vi "Save data file (pass-fail) v5.vi"(8 "Input Cluster":T1, 11 "panel id":string) -> (0 "network file save error":errorcluster, 3 "file save path":string)   [LabVIEW 2017]
uses:
  Global 1.vi
  Global display 2.vi
  Global display 3.vi
  <vilib>/Utility/file.llb/Write Delimited Spreadsheet (string).vi
panel:
  out "Fail File path":path
  out "x != y?":bool
  out "mail file":bool
  out "Report path c drive":path
  out "Report path network":path
  out "status":string
  out "C drive root path":string
  out "network file dir path":path
  out "network dir":string
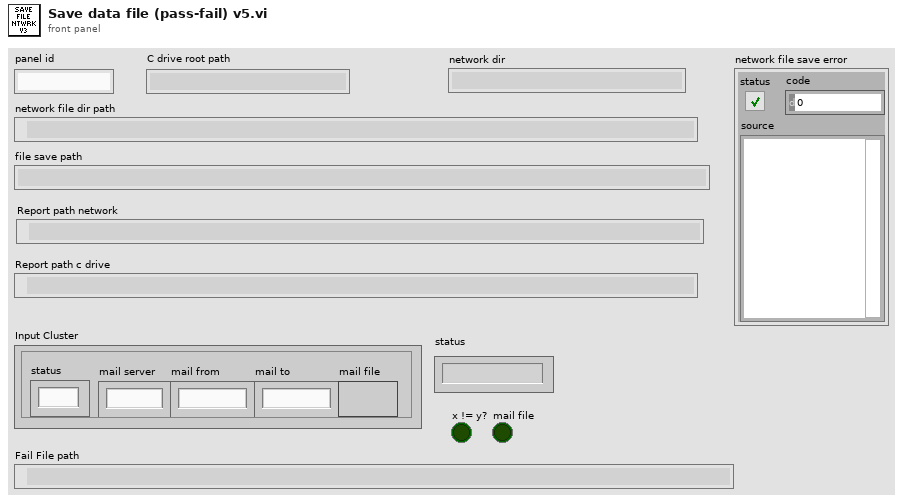
[diagram p1: front panel]
types:
  T1 = cluster{"status":string, "mail server":string, "mail from":string, "mail to":string, "mail file":bool}
  T2 = cluster{"CYCLE":dbl, "MINS":dbl, "STATUS":string}
  T3 = cluster{"NAME":string, "DESCRIPTION":string, "CYCLES":dbl, "T-RISE mins":dbl, "T-RISE deg C":dbl}
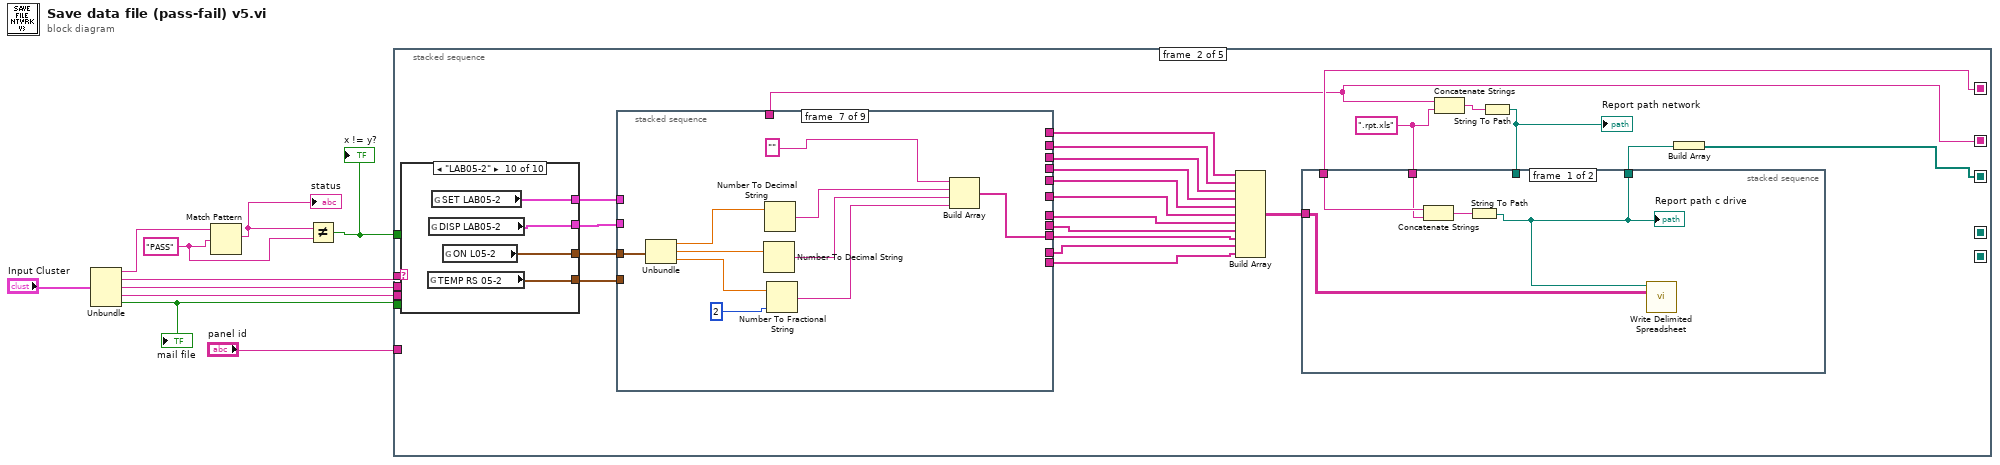
[diagram p0: block diagram]
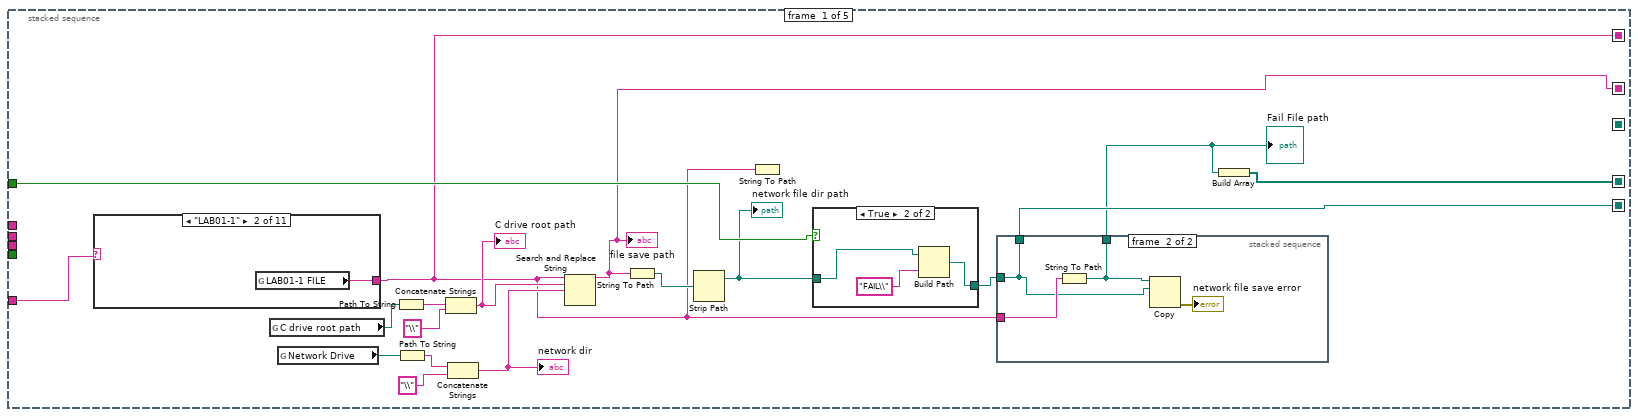
[diagram p2: hidden frame]
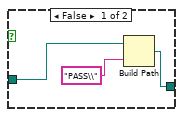
[diagram p3: hidden frame]
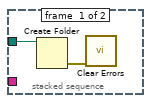
[diagram p4: hidden frame]
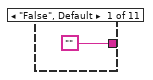
[diagram p5: hidden frame]
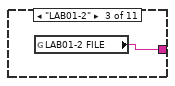
[diagram p6: hidden frame]
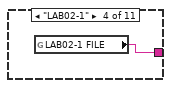
[diagram p7: hidden frame]
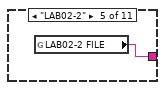
[diagram p8: hidden frame]
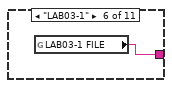
[diagram p9: hidden frame]
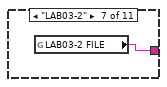
[diagram p10: hidden frame]
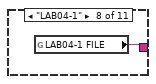
[diagram p11: hidden frame]
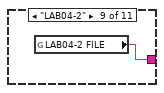
[diagram p12: hidden frame]
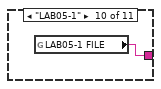
[diagram p13: hidden frame]
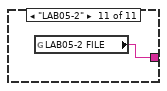
[diagram p14: hidden frame]
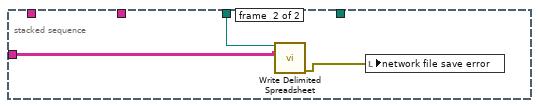
[diagram p15: hidden frame]
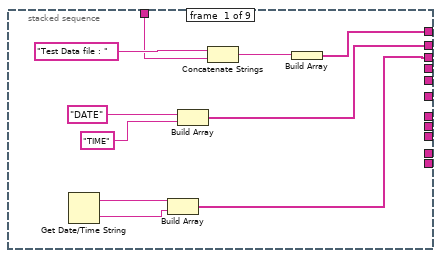
[diagram p16: hidden frame]
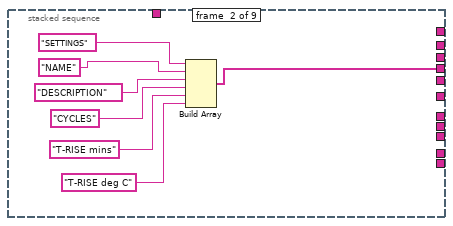
[diagram p17: hidden frame]
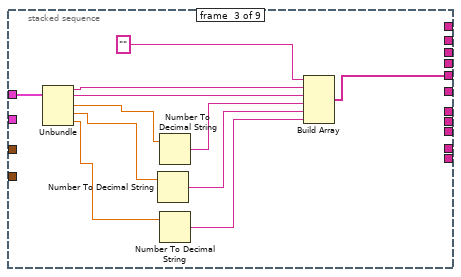
[diagram p18: hidden frame]
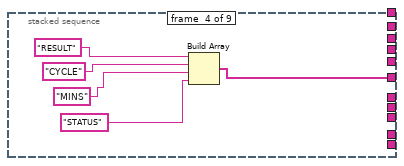
[diagram p19: hidden frame]
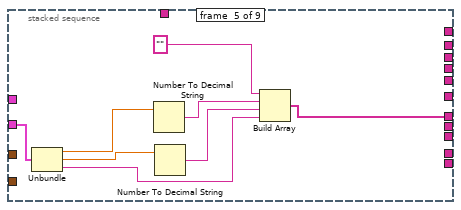
[diagram p20: hidden frame]
diagram:
  w10 = "PASS"
  n1 = Unbundle("Input Cluster") -> ("status"=w8:string, "mail server"=w2:string, "mail from"=w3:string, "mail to"=w4:string, "mail file"=w5:bool)
  "mail file" <- w5
  n2 = Match Pattern(string=w8, regular expression=w10) -> (match substring=w9:string)  [unwired: 1 in, 3 out]
  "status" <- w9
  n3 = Not Equal?(x=w9, y=w10) -> (x != y?=w6:bool)
  "x != y?" <- w6
  n4 = stacked-sequence {
    seq-local: [w11 _ _ _ _] -> [_ _ _ w197 _]
    seq-local: [w17 _ _ _ _] -> [_ _ _ _ _]
    seq-local: [w16 _ _ _ _] -> [_ w53 _ _ _]
    seq-local: [_ w56 _ _ _] -> [_ _ _ _ w207]
    seq-local: [w13 _ _ _ _] -> [_ w55 _ _ _]
    tunnel: w6 -> [w20 _ _ w196 _]
    tunnel: w5 -> [_ _ _ w195 _]
    tunnel: w4 -> [_ _ _ w194 _]
    tunnel: w3 -> [_ _ _ w193 w209]
    tunnel: w2 -> [_ _ _ w192 w208]
    tunnel: "panel id" -> [w15 w70 _ _ _]
    frame #0 {
      n5 = case shown="\"LAB01-1\"" w15 {
        tunnel: ["" w42 w43 w44 w45 w46 w47 w48 w49 w50 w51] -> w13
        frame "False", Default {
        }
        frame "LAB01-1" {
          n6 = global read "Global 1.vi" "LAB01-1 FILE"() -> (w42:string)
        }
        frame "LAB01-2" {
          n7 = global read "Global 1.vi" "LAB01-2 FILE"() -> (w43:string)
        }
        frame "LAB02-1" {
          n8 = global read "Global 1.vi" "LAB02-1 FILE"() -> (w44:string)
        }
        frame "LAB02-2" {
          n9 = global read "Global 1.vi" "LAB02-2 FILE"() -> (w45:string)
        }
        frame "LAB03-1" {
          n10 = global read "Global 1.vi" "LAB03-1 FILE"() -> (w46:string)
        }
        frame "LAB03-2" {
          n11 = global read "Global 1.vi" "LAB03-2 FILE"() -> (w47:string)
        }
        frame "LAB04-1" {
          n12 = global read "Global 1.vi" "LAB04-1 FILE"() -> (w48:string)
        }
        frame "LAB04-2" {
          n13 = global read "Global 1.vi" "LAB04-2 FILE"() -> (w49:string)
        }
        frame "LAB05-1" {
          n14 = global read "Global 1.vi" "LAB05-1 FILE"() -> (w50:string)
        }
        frame "LAB05-2" {
          n15 = global read "Global 1.vi" "LAB05-2 FILE"() -> (w51:string)
        }
      }
      n16 = global read "Global 1.vi" "C drive root path"() -> (w22:path)
      n17 = global read "Global 1.vi" "Network Drive"() -> (w28:path)
      n18 = Path To String(path=w22) -> (string=w23:string)
      n19 = Path To String(path=w28) -> (string=w27:string)
      n20 = Concatenate Strings(w23, "\\") -> (w21:string)
      "C drive root path" <- w21
      n21 = Concatenate Strings(w27, "\\") -> (w25:string)
      "network dir" <- w25
      n22 = Search and Replace String(input string=w13, search string=w21, replace string=w25) -> (result string=w16:string)  [unwired: 5 in, 3 out]
      "file save path" <- w16
      n23 = String To Path(string=w16) -> (path=w14:path)
      n24 = Strip Path(path=w14) -> (stripped path=w18:path)  [unwired: 1 out]
      "network file dir path" <- w18
      n25 = String To Path(string=w13) -> ()  [unwired: 1 out]
      n26 = case shown="True" w20 {
        tunnel: [w29 w34] -> w19
        tunnel: w18 -> [w30 w32]
        frame False {
          n27 = Build Path(base path=w30, name or relative path="PASS\\") -> (appended path=w29:path)
        }
        frame True {
          n28 = Build Path(base path=w32, name or relative path="FAIL\\") -> (appended path=w34:path)
        }
      }
      n29 = stacked-sequence {
        tunnel: w19 -> [w36 w38]
        tunnel: w13 -> [_ w39]
        tunnel: [_ w38] -> w17
        tunnel: [_ w37] -> w12
        frame #0 {
          n30 = Create Folder(path (use dialog)=w36) -> (error out=w35:errorcluster)  [unwired: 2 in, 2 out]
          n31 = call <vilib>:"Clear Errors.vi"("error in (no error)"=w35) -> ()  [unwired: 5 in, 2 out]
        }
        frame #1 {
          n32 = String To Path(string=w39) -> (path=w37:path)
          n33 = Copy(10:w38, 11:w37) -> (0:→"network file save error":errorcluster)  [unwired: 3 in, 2 out]
        }
      }
      "Fail File path" <- w12
      n34 = Build Array(w12) -> (w11:path[])
    }
    frame #1 {
      w54 = ".rpt.xls"
      n35 = case shown="\"LAB05-2\"" w70 {
        tunnel: [w154 w158 w162 w166 w170 w174 w178 w182 w186 w190] -> w75
        tunnel: [w153 w157 w161 w165 w169 w173 w177 w181 w185 w189] -> w74
        tunnel: [w152 w156 w160 w164 w168 w172 w176 w180 w184 w188] -> w73
        tunnel: [w151 w155 w159 w163 w167 w171 w175 w179 w183 w187] -> w72
        frame "LAB01-1", Default {
          n36 = global read "Global display 3.vi" "TEMP RS 01-1"() -> (w151:cluster{"TL":dbl, "TN":dbl})
          n37 = global read "Global display 2.vi" "DISP LAB01-1"() -> (w153:T2)
          n38 = global read "Global display 2.vi" "SET LAB01-1"() -> (w154:T3)
          n39 = global read "Global display 2.vi" "ON L01-1"() -> (w152:cluster{"amps":dbl, "volts":dbl, "pf":dbl})
        }
        frame "LAB01-2" {
          n40 = global read "Global display 3.vi" "TEMP RS 01-2"() -> (w155:cluster{"TL":dbl, "TN":dbl})
          n41 = global read "Global display 2.vi" "DISP LAB01-2"() -> (w157:T2)
          n42 = global read "Global display 2.vi" "SET LAB01-2"() -> (w158:T3)
          n43 = global read "Global display 2.vi" "ON L01-2"() -> (w156:cluster{"amps":dbl, "volts":dbl, "pf":dbl})
        }
        frame "LAB02-1" {
          n44 = global read "Global display 3.vi" "TEMP RS 02-1"() -> (w159:cluster{"TL":dbl, "TN":dbl})
          n45 = global read "Global display 2.vi" "DISP LAB02-1"() -> (w161:T2)
          n46 = global read "Global display 2.vi" "SET LAB02-1"() -> (w162:T3)
          n47 = global read "Global display 2.vi" "ON L02-1"() -> (w160:cluster{"amps":dbl, "volts":dbl, "pf":dbl})
        }
        frame "LAB02-2" {
          n48 = global read "Global display 3.vi" "TEMP RS 02-2"() -> (w163:cluster{"TL":dbl, "TN":dbl})
          n49 = global read "Global display 2.vi" "DISP LAB02-2"() -> (w165:T2)
          n50 = global read "Global display 2.vi" "SET LAB02-2"() -> (w166:T3)
          n51 = global read "Global display 2.vi" "ON L02-2"() -> (w164:cluster{"amps":dbl, "volts":dbl, "pf":dbl})
        }
        frame "LAB03-1" {
          n52 = global read "Global display 3.vi" "TEMP RS 03-1"() -> (w167:cluster{"TL":dbl, "TN":dbl})
          n53 = global read "Global display 2.vi" "DISP LAB03-1"() -> (w169:T2)
          n54 = global read "Global display 2.vi" "SET LAB03-1"() -> (w170:T3)
          n55 = global read "Global display 2.vi" "ON L03-1"() -> (w168:cluster{"amps":dbl, "volts":dbl, "pf":dbl})
        }
        frame "LAB03-2" {
          n56 = global read "Global display 3.vi" "TEMP RS 03-2"() -> (w171:cluster{"TL":dbl, "TN":dbl})
          n57 = global read "Global display 2.vi" "DISP LAB03-2"() -> (w173:T2)
          n58 = global read "Global display 2.vi" "SET LAB03-2"() -> (w174:T3)
          n59 = global read "Global display 2.vi" "ON L03-2"() -> (w172:cluster{"amps":dbl, "volts":dbl, "pf":dbl})
        }
        frame "LAB04-1" {
          n60 = global read "Global display 3.vi" "TEMP RS 04-1"() -> (w175:cluster{"TL":dbl, "TN":dbl})
          n61 = global read "Global display 2.vi" "DISP LAB04-1"() -> (w177:T2)
          n62 = global read "Global display 2.vi" "SET LAB04-1"() -> (w178:T3)
          n63 = global read "Global display 2.vi" "ON L04-1"() -> (w176:cluster{"amps":dbl, "volts":dbl, "pf":dbl})
        }
        frame "LAB04-2" {
          n64 = global read "Global display 3.vi" "TEMP RS 04-2"() -> (w179:cluster{"TL":dbl, "TN":dbl})
          n65 = global read "Global display 2.vi" "DISP LAB04-2"() -> (w181:T2)
          n66 = global read "Global display 2.vi" "SET LAB04-2"() -> (w182:T3)
          n67 = global read "Global display 2.vi" "ON L04-2"() -> (w180:cluster{"amps":dbl, "volts":dbl, "pf":dbl})
        }
        frame "LAB05-1" {
          n68 = global read "Global display 3.vi" "TEMP RS 05-1"() -> (w183:cluster{"TL":dbl, "TN":dbl})
          n69 = global read "Global display 2.vi" "DISP LAB05-1"() -> (w185:T2)
          n70 = global read "Global display 2.vi" "SET LAB05-1"() -> (w186:T3)
          n71 = global read "Global display 2.vi" "ON L05-1"() -> (w184:cluster{"amps":dbl, "volts":dbl, "pf":dbl})
        }
        frame "LAB05-2" {
          n72 = global read "Global display 3.vi" "TEMP RS 05-2"() -> (w187:cluster{"TL":dbl, "TN":dbl})
          n73 = global read "Global display 2.vi" "DISP LAB05-2"() -> (w189:T2)
          n74 = global read "Global display 2.vi" "SET LAB05-2"() -> (w190:T3)
          n75 = global read "Global display 2.vi" "ON L05-2"() -> (w188:cluster{"amps":dbl, "volts":dbl, "pf":dbl})
        }
      }
      n76 = stacked-sequence {
        tunnel: w75 -> [_ _ w111 _ _ _ _ _ _]
        tunnel: w74 -> [_ _ _ _ w124 _ _ _ _]
        tunnel: w73 -> [_ _ _ _ _ _ w139 _ _]
        tunnel: w72 -> [_ _ _ _ _ _ _ _ w150]
        tunnel: [_ w94 _ _ _ _ _ _ _] -> w66
        tunnel: [_ _ w101 _ _ _ _ _ _] -> w65
        tunnel: [_ _ _ w112 _ _ _ _ _] -> w64
        tunnel: [_ _ _ _ w117 _ _ _ _] -> w63
        tunnel: [_ _ _ _ _ w125 _ _ _] -> w62
        tunnel: [_ _ _ _ _ _ w133 _ _] -> w61
        tunnel: [_ _ _ _ _ _ _ w140 _] -> w60
        tunnel: [_ _ _ _ _ _ _ _ w144] -> w59
        tunnel: [w91 _ _ _ _ _ _ _ _] -> w69
        tunnel: [w88 _ _ _ _ _ _ _ _] -> w68
        tunnel: [w85 _ _ _ _ _ _ _ _] -> w67
        tunnel: w53 -> [w84 _ _ _ _ _ _ _ _]
        frame #0 {
          n77 = Get Date/Time String() -> (date string=w87:string, time string=w86:string)  [unwired: 3 in]
          n78 = Build Array(w87, w86) -> (w85:string[])
          n79 = Build Array("DATE", "TIME") -> (w88:string[])
          n80 = Concatenate Strings("Test Data file : ", w84) -> (w92:string)
          n81 = Build Array(w92) -> (w91:string[])
        }
        frame #1 {
          n82 = Build Array("SETTINGS", "NAME", "DESCRIPTION", "CYCLES", "T-RISE mins", "T-RISE deg C") -> (w94:string[])
        }
        frame #2 {
          n83 = Unbundle(w111) -> ("NAME"=w106:string, "DESCRIPTION"=w105:string, "CYCLES"=w110:dbl, "T-RISE mins"=w109:dbl, "T-RISE deg C"=w108:dbl)
          n84 = Number To Decimal String(number=w109) -> (decimal integer string=w103:string)  [unwired: 1 in]
          n85 = Number To Decimal String(number=w110) -> (decimal integer string=w104:string)  [unwired: 1 in]
          n86 = Number To Decimal String(number=w108) -> (decimal integer string=w102:string)  [unwired: 1 in]
          n87 = Build Array("", w106, w105, w104, w103, w102) -> (w101:string[])
        }
        frame #3 {
          n88 = Build Array("RESULT", "CYCLE", "MINS", "STATUS") -> (w112:string[])
        }
        frame #4 {
          n89 = Unbundle(w124) -> ("CYCLE"=w123:dbl, "MINS"=w122:dbl, "STATUS"=w118:string)
          n90 = Number To Decimal String(number=w123) -> (decimal integer string=w120:string)  [unwired: 1 in]
          n91 = Number To Decimal String(number=w122) -> (decimal integer string=w119:string)  [unwired: 1 in]
          n92 = Build Array("", w120, w119, w118) -> (w117:string[])
        }
        frame #5 {
          n93 = Build Array("TEST", "AMPS", "VOLTS", "PF") -> (w125:string[])
        }
        frame #6 {
          n94 = Unbundle(w139) -> ("amps"=w138:dbl, "volts"=w137:dbl, "pf"=w132:dbl)
          n95 = Number To Decimal String(number=w137) -> (decimal integer string=w134:string)  [unwired: 1 in]
          n96 = Number To Decimal String(number=w138) -> (decimal integer string=w135:string)  [unwired: 1 in]
          n97 = Number To Fractional String(number=w132, precision (6)=2) -> (F-format string=w131:string)  [unwired: 2 in]
          n98 = Build Array("", w135, w134, w131) -> (w133:string[])
        }
        frame #7 {
          n99 = Build Array("TEMP RISE", "LIVE", "NEUTRAL") -> (w140:string[])
        }
        frame #8 {
          n100 = Unbundle(w150) -> ("TL"=w149:dbl, "TN"=w148:dbl)
          n101 = Number To Decimal String(number=w149) -> (decimal integer string=w146:string)  [unwired: 1 in]
          n102 = Number To Decimal String(number=w148) -> (decimal integer string=w145:string)  [unwired: 1 in]
          n103 = Build Array("", w146, w145) -> (w144:string[])
        }
      }
      n104 = Build Array(w69, w68, w67, w66, w65, w64, w63, w62, w61, w60, w59) -> (w58:string[][])
      n105 = Concatenate Strings(w53, w54) -> (w71:string)
      n106 = String To Path(string=w71) -> (path=w57:path)
      "Report path network" <- w57
      n107 = stacked-sequence {
        tunnel: w58 -> [w76 w82]
        tunnel: w57 -> [_ w83]
        tunnel: w55 -> [w80 _]
        tunnel: w54 -> [w79 _]
        tunnel: [w77 _] -> w52
        frame #0 {
          n108 = Concatenate Strings(w80, w79) -> (w78:string)
          n109 = String To Path(string=w78) -> (path=w77:path)
          "Report path c drive" <- w77
          n110 = call-poly <vilib>:"Write Delimited Spreadsheet.vi"("file path (dialog if empty)"=w77, "2D data"=w76) -> ()  [unwired: 12 in, 2 out]
        }
        frame #1 {
          n111 = call-poly <vilib>:"Write Delimited Spreadsheet.vi"("file path (dialog if empty)"=w83, "2D data"=w82) -> ("error out"=w81:errorcluster)  [unwired: 12 in, 1 out]
          n112 = local write "network file save error"(w81) -> ()
        }
      }
      n113 = Build Array(w52) -> (w56:path[])
    }
    frame #2 {
      n114 = Wait (ms)(milliseconds to wait=500) -> ()  [unwired: 1 out]
    }
    frame #3 {
      # "mail test fail file"
      n115 = And(x=w196, y=w195) -> (x .and. y?=w198:bool)
      n116 = case shown="True" w198 {
        tunnel: w197 -> [_ w199]
        tunnel: w194 -> [_ w203]
        tunnel: w193 -> [_ w202]
        tunnel: w192 -> [_ w201]
        frame False {
        }
        frame True {
          w200 = "TEST FAIL FILE"
          n117 = call "sub vi - send mail with attach v4.vi"("TO:"=w203, "subject"=w200, "Info"=w200, "from"=w202, "out going server"=w201, "Attachements"=w199) -> ("error out"=w204:errorcluster)  [unwired: 9 in]
          n118 = local write "network file save error"(w204) -> ()
        }
      }
    }
    frame #4 {
      w205 = "Lab Panel Test Report "
      # "mail test report"
      n119 = global read "Global display 2.vi" "Mail test file to:"() -> (w210:string)
      n120 = call "sub vi - send mail with attach v4.vi"("TO:"=w210, "subject"=w205, "Info"=w205, "from"=w209, "out going server"=w208, "Attachements"=w207) -> ("error out"=w206:errorcluster)  [unwired: 9 in]
      n121 = local write "network file save error"(w206) -> ()
    }
  }
